vi "Pick and place sequence.vi"(6 "Component Tray map":dbl[][](array[numeric]), 8 "error in (no error)":errorcluster, 9 "Assembly Tray map":dbl[][](array[numeric]), 10 "PUT map":dbl[][](array[numeric]), 11 "Assembly Run in":refnum<class "Assembly Run.lvclass">) -> (0 "error out":errorcluster, 3 "Assembly Run out":refnum<class "Assembly Run.lvclass">)   [LabVIEW 2020, in "Assembly Run.lvclass"]
uses:
  Assembly Run.lvclass
  Workspace/Fixture Enum.ctl
  Workspace/Fixture.lvclass
  Routine/Routine Enum.ctl
  Routine/Routine.lvclass
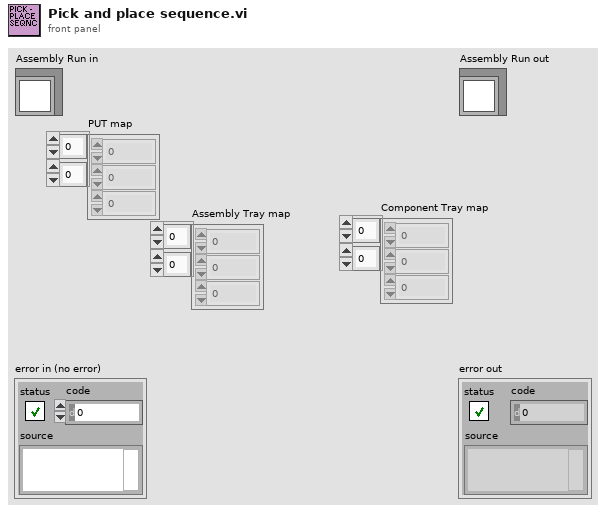
[diagram p1: front panel]
types:
  T1 = typedef "Routine.lvclass/Routine Enum.ctl" = enum16{"Primary Pick Up", "Pick Up All", "Put Down Secondary", "Put Down All", "Release Syringe", "Secondary Pick Up", "Secure Syringe", "Dispense on Plate", "Dispense on Kapton", "Dispense on Sensor"}
  T2 = typedef "Fixture.lvclass/Fixture Enum.ctl" = enum16{"Assembly Tray", "Syringe Space", "Component", "Pick Up Tool", "Current Position"}
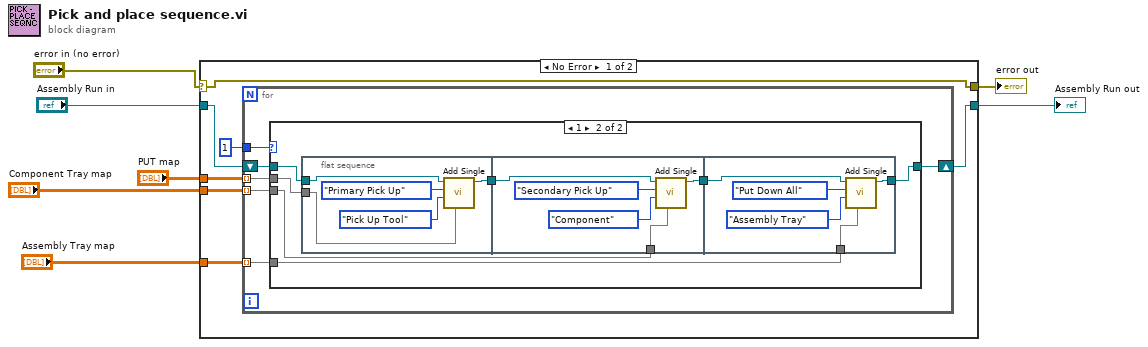
[diagram p0: block diagram]
diagram:
  n1 = case shown="No Error" "error in (no error)" {
    selector: "error in (no error)" -> [w14 w45]
    tunnel: [w14 w45] -> w6
    tunnel: [w11 w44] -> w4
    tunnel: "Assembly Run in" -> [w12 w44]
    tunnel: "PUT map" -> [w10 _]
    tunnel: "Component Tray map" -> [w9 _]
    tunnel: "Assembly Tray map" -> [w8 _]
    frame No Error {
      n2 = for {
        tunnel: 1 -> [w18]
        shift-right: [w20] -> w11
        shift-left: w12 -> [w19]
        tunnel: w10 -> [w17] mode=indexing
        tunnel: w9 -> [w16] mode=indexing
        tunnel: w8 -> [w15] mode=indexing
        n3 = case shown="1" w18 {
          tunnel: [w21 w28] -> w20
          tunnel: w19 -> [w21 w27]
          tunnel: w17 -> [_ w24]
          tunnel: w16 -> [_ w23]
          tunnel: w15 -> [_ w22]
          frame 0, Default {
          }
          frame 1 {
            n4 = flat-sequence {
              tunnel: w27 -> [w32]
              tunnel: [w33] -> w26
              tunnel: w24 -> [w31]
              tunnel: w26 -> [w38]
              tunnel: [w37] -> w25
              tunnel: w23 -> [w36]
              tunnel: [w42] -> w28
              tunnel: w25 -> [w43]
              tunnel: w22 -> [w41]
              frame #0 {
                n5 = call-dynamic "Add Single.vi"("Gantry map"=w31, "Fixture"=Fixture_Enum."Pick Up Tool", "Routine"=Routine_Enum."Primary Pick Up" ("Routine 2"), "UI in"=w32) -> ("UI out"=w33:refnum<class "Assembly Run.lvclass">)  [unwired: 5 in, 1 out]
              }
              frame #1 {
                n6 = call-dynamic "Add Single.vi"("Gantry map"=w36, "Fixture"=Fixture_Enum."Component", "Routine"=Routine_Enum."Secondary Pick Up" ("Routine 2"), "UI in"=w38) -> ("UI out"=w37:refnum<class "Assembly Run.lvclass">)  [unwired: 5 in, 1 out]
              }
              frame #2 {
                n7 = call-dynamic "Add Single.vi"("Gantry map"=w41, "Fixture"=Fixture_Enum."Assembly Tray", "Routine"=Routine_Enum."Put Down All" ("Routine 2"), "UI in"=w43) -> ("UI out"=w42:refnum<class "Assembly Run.lvclass">)  [unwired: 5 in, 1 out]
              }
            }
          }
        }
      }
    }
    frame Error {
    }
  }
  "error out" <- w6
  "Assembly Run out" <- w4
